vi "Initialize Module.vi"(8 "error in":errorcluster, 11 "module in":refnum<class "Module.lvclass">) -> (0 "error out":errorcluster, 3 "module out":refnum<class "Module.lvclass">)   [LabVIEW 2017, in "Scan Engine Scripting.lvlib" / "Module.lvclass"]
uses:
  Module.lvclass
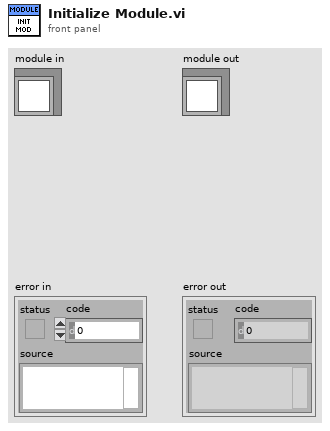
[diagram p1: front panel]
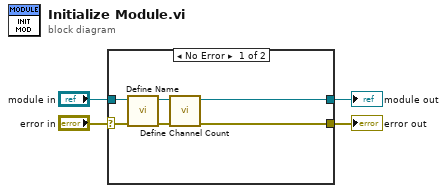
[diagram p0: block diagram]
diagram:
  n1 = case shown="No Error" "error in" {
    selector: "error in" -> [w8 w12]
    tunnel: [w6 w12] -> w3
    tunnel: [w5 w11] -> w1
    tunnel: "module in" -> [w10 w11]
    frame No Error {
      n2 = call-dynamic "Define Name.vi"("error in"=w8, "Module in"=w10) -> ("error out"=w7:errorcluster, "Module out"=w9:refnum<class "Module.lvclass">)  [unwired: 8 in]
      n3 = call-dynamic "Define Channel Count.vi"("error in"=w7, "Module in"=w9) -> ("error out"=w6:errorcluster, "Module out"=w5:refnum<class "Module.lvclass">)  [unwired: 8 in]
    }
    frame Error {
    }
  }
  "error out" <- w3
  "module out" <- w1
